vi "TestExec.Send Funct RTN Data.vi"(6 "SkipRtn":bool, 8 "Error":errorcluster, 9 "RTN Route (Data2)":variant, 10 "RTN Data":T1 {"MeasData"."Status" items=["LOG", "PASS", "FAIL", "ERROR"]; "Attr"."Status" items=["LOG", "PASS", "FAIL", "ERROR"]; "Num"."Status" items=["LOG", "PASS", "FAIL", "ERROR"]}, 11 "Q In":refnum<queue>) -> (0 "error out":errorcluster)   [LabVIEW 2024]
uses:
  <vilib>/KATE/Queues/Q.Element.ctl
  TestExec.Local Result Data.ctl
  Results/Result.Attribute.ctl
  Results/Result.Measurement and Attribute Item Status.ctl
  Results/Result.Numeric.ctl
  Results/Result.Limit Type.ctl
  Results/Result XML/TestResult.SW Item.ctl
  Reports/Report.Result FileDataObject.ctl
  Results/Result.Measurement Item.ctl
  <vilib>/KATE/Queues/Queue Utils.lvlib
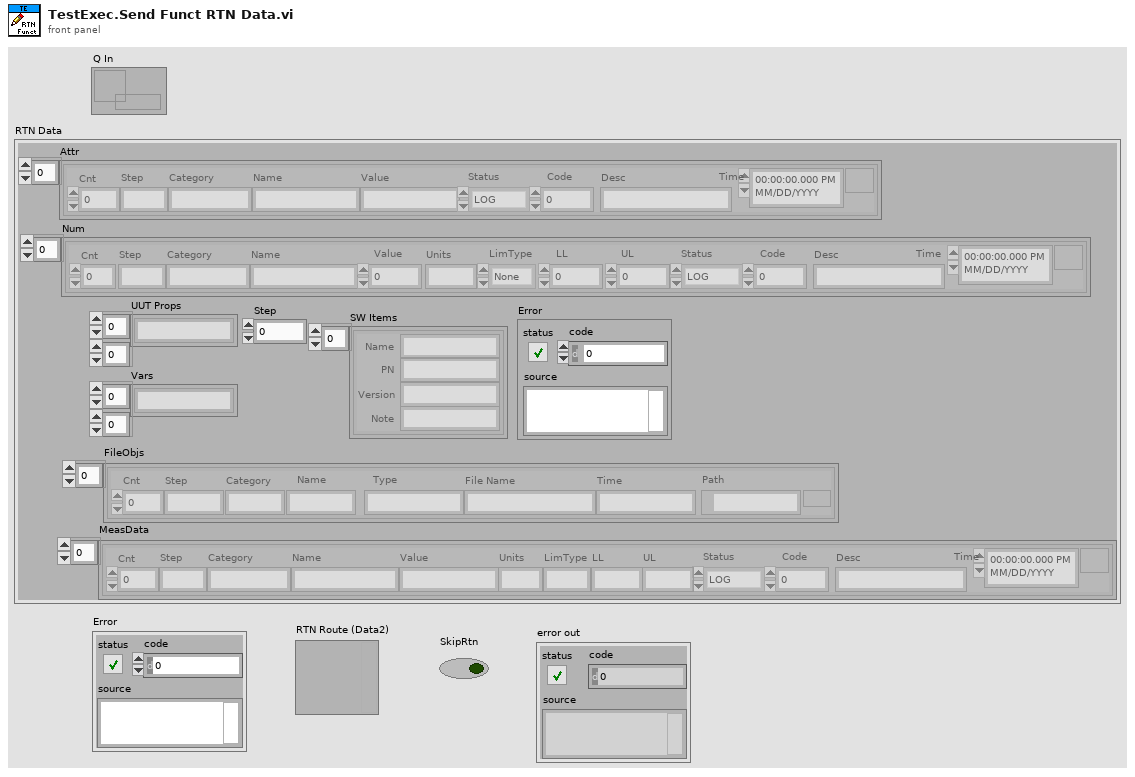
[diagram p1: front panel]
types:
  T1 = typedef "TestExec.Local Result Data.ctl" = cluster{"Attr":T2[], "Num":T4[], "UUT Props":string[][], "Vars":string[][], "SW Items":T6[], "Error":errorcluster, "Step":i32, "FileObjs":T7[], "MeasData":T8[]}
  T2 = typedef "Result.Attribute.ctl" = cluster{"Cnt":i32, "Step":string, "Category":string, "Name":string, "Value":string, "Status":T3, "Code":i32, "Desc":string, "Time":timestamp}
  T3 = typedef "Result.Measurement and Attribute Item Status.ctl" = i32
  T4 = typedef "Result.Numeric.ctl" = cluster{"Cnt":i32, "Step":string, "Category":string, "Name":string, "Value":dbl, "Units":string, "LimType":T5, "LL":dbl, "UL":dbl, "Status":T3, "Code":i32, "Desc":string, "Time":timestamp}
  T5 = typedef "Result.Limit Type.ctl" = enum16{"None", "EQ", "NE", "GT", "LT", "GE", "LE", "GTLT", "GELE", "GELT", "GTLE", "LTGT", "LEGE", "LEGT", "LTGE", "Contains", "NotContains"}
  T6 = typedef "TestResult.SW Item.ctl" = cluster{"Name":string, "PN":string, "Version":string, "Note":string}
  T7 = typedef "Report.Result FileDataObject.ctl" = cluster{"Cnt":i32, "Step":string, "Category":string, "Name":string, "Type":string, "File Name":string, "Time":string, "Path":path}
  T8 = typedef "Result.Measurement Item.ctl" = cluster{"Cnt":i32, "Step":string, "Category":string, "Name":string, "Value":string, "Units":string, "LimType":string, "LL":string, "UL":string, "Status":T3, "Code":i32, "Desc":string, "Time":timestamp}
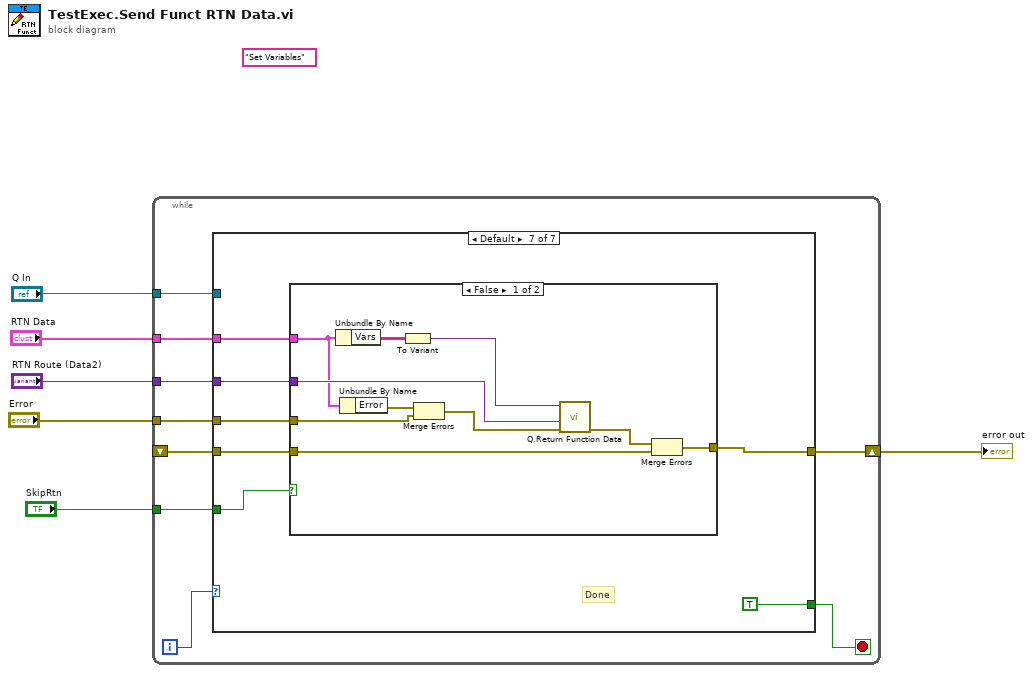
[diagram p0: block diagram]
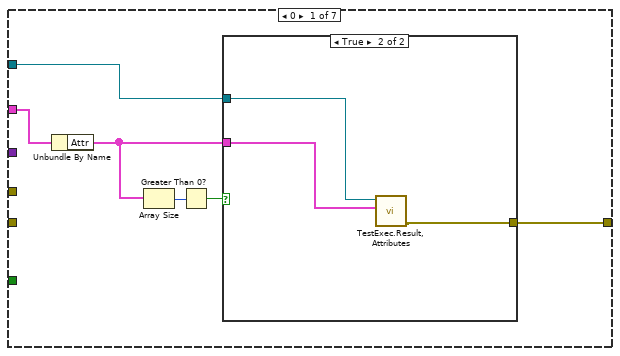
[diagram p2: hidden frame]
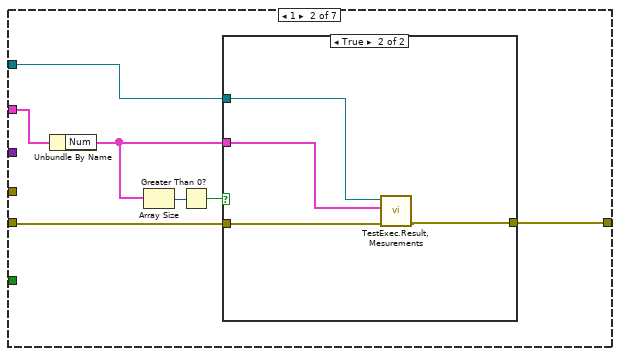
[diagram p4: hidden frame]
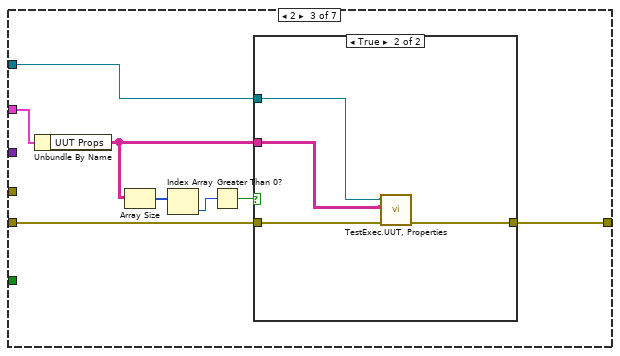
[diagram p6: hidden frame]
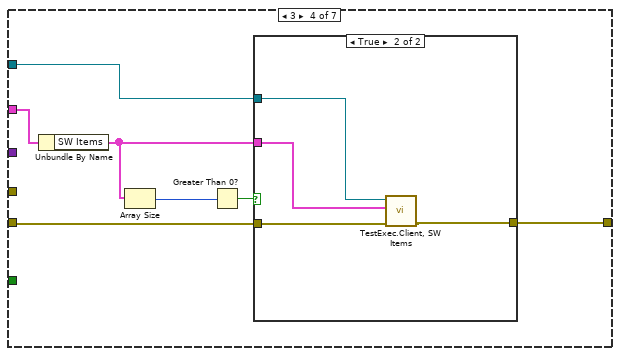
[diagram p8: hidden frame]
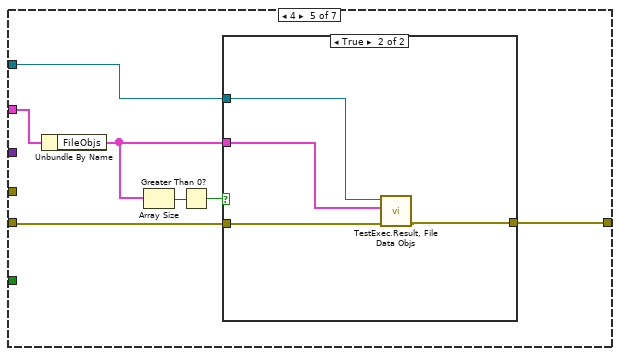
[diagram p10: hidden frame]
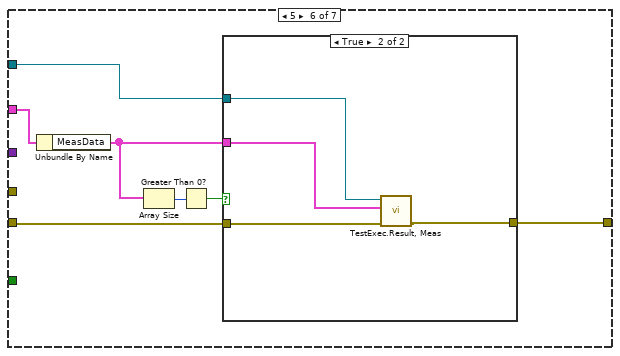
[diagram p12: hidden frame]
diagram:
  (unwired) "Set Variables" ("Cmd")
  n1 = while {
    shift-right: [w12] -> w6
    shift-left: _ -> [w13]
    tunnel: "RTN Data" -> [w11]
    tunnel: "Q In" -> [w10]
    tunnel: "RTN Route (Data2)" -> [w9]
    tunnel: "Error" -> [w8]
    tunnel: "SkipRtn" -> [w7]
    i -> [w15]
    stop <- w14 stop-if-true
    n2 = case shown="Default" w15 {
      tunnel: [_ _ _ _ _ _ TRUE] -> w14
      tunnel: w13 -> [_ w25 w36 w48 w59 w70 w85]
      tunnel: [w17 w27 w40 w51 w61 w72 w84] -> w12
      tunnel: w11 -> [w21 w31 w43 w54 w65 w76 w83]
      tunnel: w10 -> [w16 w26 w39 w50 w60 w71 _]
      tunnel: w9 -> [_ _ _ _ _ _ w86]
      tunnel: w8 -> [_ _ _ _ _ _ w82]
      tunnel: w7 -> [_ _ _ _ _ _ w81]
      frame 0 {
        n3 = Unbundle By Name(w21) -> ("Attr"=w18:T2[])
        n4 = Array Size(array=w18) -> (size(s)=w19:i32)
        n5 = Greater Than 0?(x=w19) -> (x > 0?=w20:bool)
        n6 = case shown="True" w20 {
          tunnel: w18 -> [_ w23]
          tunnel: [_ w22] -> w17
          tunnel: w16 -> [_ w24]
          frame False {
          }
          frame True {
            n7 = call "TestExec.Result, Attributes.vi"("Attributes"=w23, "Q In"=w24) -> ("error out"=w22:errorcluster)  [unwired: 9 in]
          }
        }
      }
      frame 1 {
        n8 = Unbundle By Name(w31) -> ("Num"=w28:T4[])
        n9 = Array Size(array=w28) -> (size(s)=w29:i32)
        n10 = Greater Than 0?(x=w29) -> (x > 0?=w30:bool)
        n11 = case shown="True" w30 {
          tunnel: w28 -> [_ w34]
          tunnel: [_ w33] -> w27
          tunnel: w26 -> [_ w35]
          tunnel: w25 -> [_ w32]
          frame False {
          }
          frame True {
            n12 = call "TestExec.Result, Mesurements.vi"("error in"=w32, "Numeric"=w34, "Q In"=w35) -> ("error out"=w33:errorcluster)  [unwired: 8 in]
          }
        }
      }
      frame 2 {
        n13 = Unbundle By Name(w43) -> ("UUT Props"=w41:string[][])
        n14 = Array Size(array=w41) -> (size(s)=w38:i32[])
        n15 = Index Array(array=w38) -> (element=w37:i32)  [unwired: 1 in]
        n16 = Greater Than 0?(x=w37) -> (x > 0?=w42:bool)
        n17 = case shown="True" w42 {
          tunnel: w41 -> [_ w46]
          tunnel: [_ w45] -> w40
          tunnel: w39 -> [_ w47]
          tunnel: w36 -> [_ w44]
          frame False {
          }
          frame True {
            n18 = call "TestExec.UUT, Properties.vi"("error in"=w44, "UUT Properties"=w46, "Q In"=w47) -> ("error out"=w45:errorcluster)  [unwired: 8 in]
          }
        }
      }
      frame 3 {
        n19 = Unbundle By Name(w54) -> ("SW Items"=w52:T6[])
        n20 = Array Size(array=w52) -> (size(s)=w49:i32)
        n21 = Greater Than 0?(x=w49) -> (x > 0?=w53:bool)
        n22 = case shown="True" w53 {
          tunnel: w52 -> [_ w56]
          tunnel: [_ w57] -> w51
          tunnel: w50 -> [_ w58]
          tunnel: w48 -> [_ w55]
          frame False {
          }
          frame True {
            n23 = call "TestExec.Client, SW Items.vi"("error in"=w55, "SW Items"=w56, "Q In"=w58) -> ("error out"=w57:errorcluster)  [unwired: 7 in, 1 out]
          }
        }
      }
      frame 4 {
        n24 = Unbundle By Name(w65) -> ("FileObjs"=w62:T7[])
        n25 = Array Size(array=w62) -> (size(s)=w63:i32)
        n26 = Greater Than 0?(x=w63) -> (x > 0?=w64:bool)
        n27 = case shown="True" w64 {
          tunnel: w62 -> [_ w68]
          tunnel: [_ w67] -> w61
          tunnel: w60 -> [_ w69]
          tunnel: w59 -> [_ w66]
          frame False {
          }
          frame True {
            n28 = call "TestExec.Result, File Data Objs.vi"("error in"=w66, "File Data Objs"=w68, "Q In"=w69) -> ("error out"=w67:errorcluster)  [unwired: 8 in]
          }
        }
      }
      frame 5 {
        n29 = Unbundle By Name(w76) -> ("MeasData"=w73:T8[])
        n30 = Array Size(array=w73) -> (size(s)=w74:i32)
        n31 = Greater Than 0?(x=w74) -> (x > 0?=w75:bool)
        n32 = case shown="True" w75 {
          tunnel: w73 -> [_ w79]
          tunnel: [_ w78] -> w72
          tunnel: w71 -> [_ w80]
          tunnel: w70 -> [_ w77]
          frame False {
          }
          frame True {
            n33 = call "TestExec.Result, Meas.vi"("error in"=w77, "Meas"=w79, "Q In"=w80) -> ("error out"=w78:errorcluster)  [unwired: 8 in]
          }
        }
      }
      frame Default {
        # "Done"
        n34 = case shown="False" w81 {
          tunnel: w86 -> [w97 _]
          tunnel: w85 -> [w93 w98]
          tunnel: [w92 w98] -> w84
          tunnel: w83 -> [w91 _]
          tunnel: w82 -> [w89 _]
          frame False {
            n35 = Unbundle By Name(w91) -> ("Vars"=w96:string[][])
            n36 = Unbundle By Name(w91) -> ("Error"=w90:errorcluster)
            n37 = To Variant(anything=w96) -> (Variant=w95:variant)
            n38 = Merge Errors(w90, w89) -> (w88:errorcluster)
            n39 = call <vilib>:"Q.Return Function Data.vi"("error in"=w88, "Data2"=w97, "Ret Data"=w95) -> ("error out"=w94:errorcluster)  [unwired: 8 in]
            n40 = Merge Errors(w94, w93) -> (w92:errorcluster)
          }
          frame True {
          }
        }
      }
    }
  }
  "error out" <- w6
